vi "Write Graph 1.vi"(8 "error in (no error)":errorcluster, 10 "Graph 1":refnum<vi>, 11 "OD600 in":refnum<class "OD600.lvclass">) -> (0 "error out":errorcluster, 3 "OD600 out":refnum<class "OD600.lvclass">)   [LabVIEW 2013, in "OD600.lvlib" / "OD600.lvclass"]
uses:
  OD600.lvclass
  OD600.lvclass/OD600.ctl
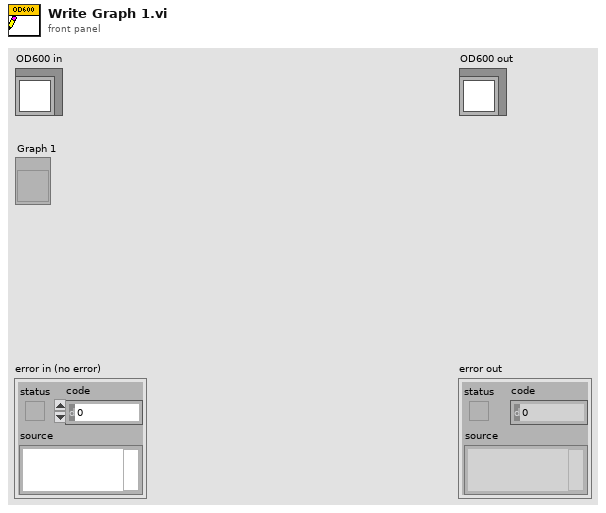
[diagram p1: front panel]
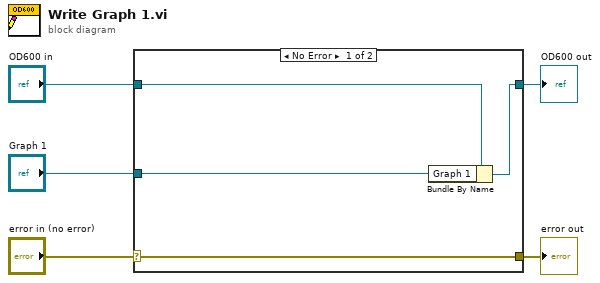
[diagram p0: block diagram]
diagram:
  n1 = case shown="No Error" "error in (no error)" {
    selector: "error in (no error)" -> [w9 w10]
    tunnel: [w9 w10] -> w4
    tunnel: [w7 w11] -> w2
    tunnel: "OD600 in" -> [w8 w11]
    tunnel: "Graph 1" -> [w6 _]
    frame No Error {
      n2 = Bundle By Name(cluster=w8, "Graph 1"=w6) -> (w7:refnum<class "OD600.lvclass">)
    }
    frame Error {
    }
  }
  "error out" <- w4
  "OD600 out" <- w2
